vi "robot - Draw Claw.vi"(4 "Diameter":dbl=10.0, 6 "Claw Angle":dbl, 7 "Claw Value":dbl=0.5, 8 "Enhance Style":bool=TRUE, 9 "Claw Color":u32(colorbox), 10 "Position":cluster{"x":dbl, "y":dbl}, 11 "Picture In":picture) -> (3 "Picture Out":picture)   [LabVIEW 2023]
doc: "This VI draws the claw for the end of the robot arm."
panel:
  in  "2nd":dbl=4.0
  in  "1st":dbl=2.5
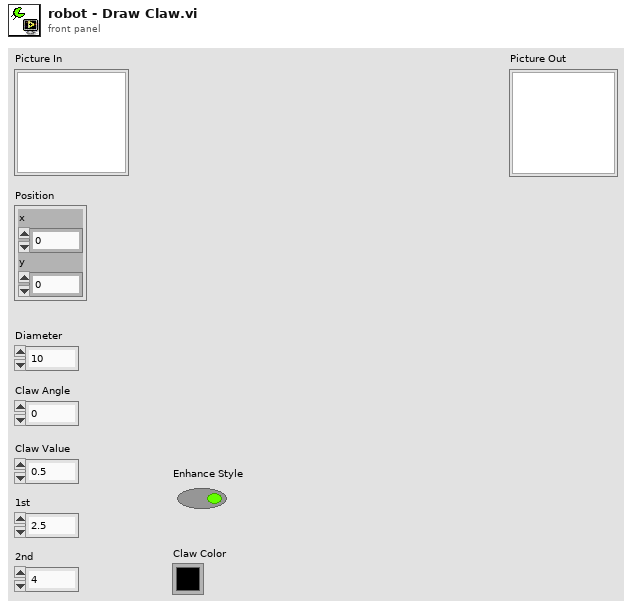
[diagram p1: front panel]
types:
  T1 = cluster{"top":dbl, "left":dbl, "height":dbl, "width":dbl}
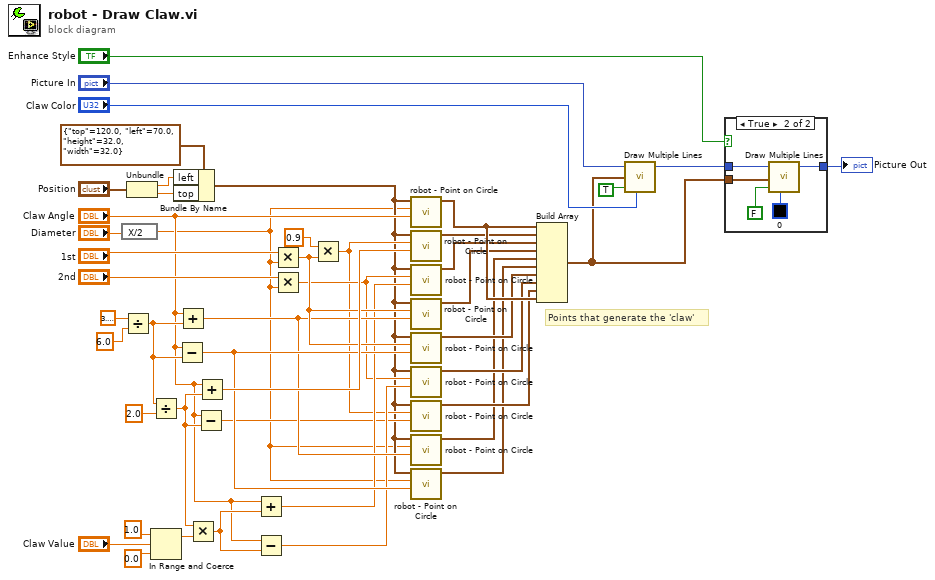
[diagram p0: block diagram]
diagram:
  # "Points that generate the 'claw'"
  n1 = expression code="X/2"("Diameter") -> (w4:dbl)
  n2 = Divide(x=3.141592653589793, y=6.0) -> (x/y=w36:dbl)
  n3 = Unbundle("Position") -> ("x"=w9:dbl, "y"=w8:dbl)
  n4 = Divide(x=w36, y=2.0) -> (x/y=w30:dbl)
  n5 = In Range and Coerce(upper limit=1.0, x="Claw Value", lower limit=0.0) -> (coerced(x)=w21:dbl)  [unwired: 1 out]
  n6 = Bundle By Name(cluster=T1 {"top"=120.0, "left"=70.0, "height"=32.0, "width"=32.0} ("Circle"), "left"=w9, "top"=w8) -> (w6:T1)
  n7 = Subtract(x="Claw Angle", y=w36) -> (x-y=w32:dbl)
  n8 = Add(x="Claw Angle", y=w36) -> (x+y=w31:dbl)
  n9 = Multiply(x=w30, y=w21) -> (x*y=w26:dbl)
  n10 = Subtract(x="Claw Angle", y=w30) -> (x-y=w7:dbl)
  n11 = Add(x="Claw Angle", y=w30) -> (x+y=w35:dbl)
  n12 = Add(x="Claw Angle", y=w26) -> (x+y=w29:dbl)
  n13 = Subtract(x="Claw Angle", y=w26) -> (x-y=w28:dbl)
  n14 = Multiply(x="1st", y=w4) -> (x*y=w33:dbl)
  n15 = Multiply(x="2nd", y=w4) -> (x*y=w27:dbl)
  n16 = Multiply(x=0.9, y=w33) -> (x*y=w24:dbl)
  n17 = call "robot - Point on Circle.vi"("Angle"="Claw Angle", "Radius"=w4, "Rect In"=w6) -> ("point"=w20:cluster{"x":dbl, "y":dbl})  [unwired: 5 in, 3 out]
  n18 = call "robot - Point on Circle.vi"("Angle"=w35, "Radius"=w24, "Rect In"=w6) -> ("point"=w19:cluster{"x":dbl, "y":dbl})  [unwired: 5 in, 3 out]
  n19 = call "robot - Point on Circle.vi"("Angle"=w29, "Radius"=w27, "Rect In"=w6) -> ("point"=w12:cluster{"x":dbl, "y":dbl})  [unwired: 5 in, 3 out]
  n20 = call "robot - Point on Circle.vi"("Angle"=w31, "Radius"=w33, "Rect In"=w6) -> ("point"=w18:cluster{"x":dbl, "y":dbl})  [unwired: 5 in, 3 out]
  n21 = call "robot - Point on Circle.vi"("Angle"=w32, "Radius"=w33, "Rect In"=w6) -> ("point"=w17:cluster{"x":dbl, "y":dbl})  [unwired: 5 in, 3 out]
  n22 = call "robot - Point on Circle.vi"("Angle"=w28, "Radius"=w27, "Rect In"=w6) -> ("point"=w15:cluster{"x":dbl, "y":dbl})  [unwired: 5 in, 3 out]
  n23 = call "robot - Point on Circle.vi"("Angle"=w7, "Radius"=w24, "Rect In"=w6) -> ("point"=w16:cluster{"x":dbl, "y":dbl})  [unwired: 5 in, 3 out]
  n24 = call "robot - Point on Circle.vi"("Angle"=w31, "Radius"=w4, "Rect In"=w6) -> ("point"=w14:cluster{"x":dbl, "y":dbl})  [unwired: 5 in, 3 out]
  n25 = call "robot - Point on Circle.vi"("Angle"=w32, "Radius"=w4, "Rect In"=w6) -> ("point"=w13:cluster{"x":dbl, "y":dbl})  [unwired: 5 in, 3 out]
  n26 = Build Array(w20, w19, w12, w18, w14, w13, w17, w15, w16, w20) -> (w40:cluster{"x":dbl, "y":dbl}[])
  n27 = call <vilib>:"Draw Multiple Lines.vi"("picture"="Picture In", "line endpoints"=w40, "fill?(F)"=TRUE, "color(black)"="Claw Color") -> ("new picture"=w41:picture)  [unwired: 5 in]
  n28 = case shown="True" "Enhance Style" {
    tunnel: w41 -> [w47 w52]
    tunnel: [w47 w51] -> w1
    tunnel: w40 -> [_ w48]
    frame False {
    }
    frame True {
      n29 = call <vilib>:"Draw Multiple Lines.vi"("picture"=w52, "line endpoints"=w48, "fill?(F)"=FALSE, "color(black)"=u32 0) -> ("new picture"=w51:picture)  [unwired: 5 in]
    }
  }
  "Picture Out" <- w1
